vi "get_target_configuration.vi"(8 "error in":errorcluster, 11 "target ref":refnum<k24>) -> (0 "error out":errorcluster, 2 "Target Configuration Data":T1, 3 "target ref out":refnum<k24>)   [LabVIEW 2020]
uses:
  controls/target_configuration_cluster.ctl
  NationalInstruments.VeriStand.SystemDefinitionAPI
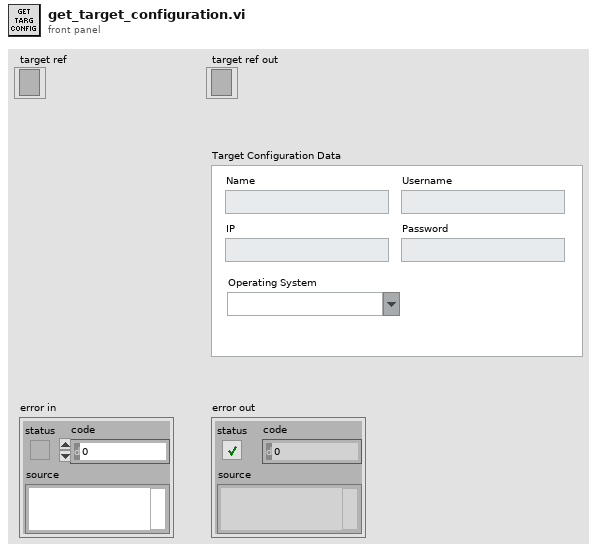
[diagram p1: front panel]
types:
  T1 = typedef "target_configuration_cluster.ctl" = cluster{"Name":string, "IP":string, "Username":string, "Password":string, "Operating System":string}
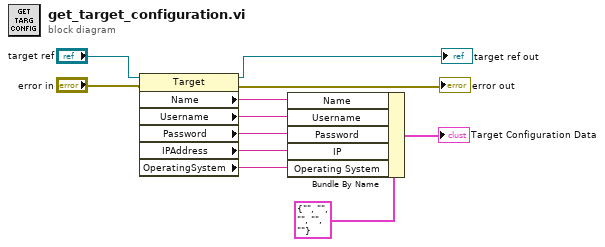
[diagram p0: block diagram]
diagram:
  n1 = property class="Target"(reference="target ref", error in="error in") -> (reference out=→"target ref out":refnum<k24>, error out=→"error out":errorcluster, "Name"=w6:string, "Username"=w5:string, "Password"=w4:string, "IPAddress"=w3:string, "OperatingSystem"=w2:string)
  n2 = Bundle By Name(cluster=T1 {"Name"="", "IP"="", "Username"="", "Password"="", "Operating System"=""} ("Target Configuration Data"), "Name"=w6, "Username"=w5, "Password"=w4, "IP"=w3, "Operating System"=w2) -> (→"Target Configuration Data":T1)
